vi "Has Documents.vi"(8 "error in (no error)":errorcluster, 11 "YAML Parser in":refnum<class "YAML Parser.lvclass">) -> (0 "error out":errorcluster, 3 "YAML Parser out":refnum<class "YAML Parser.lvclass">)   [LabVIEW 2015, in "YAML Parser.lvclass"]
uses:
  YAML Parser.lvclass
  <vilib>/regexp/Match Regular Expression.xnode
panel:
  out "Documents Count":i32
  out "Has Documents":bool
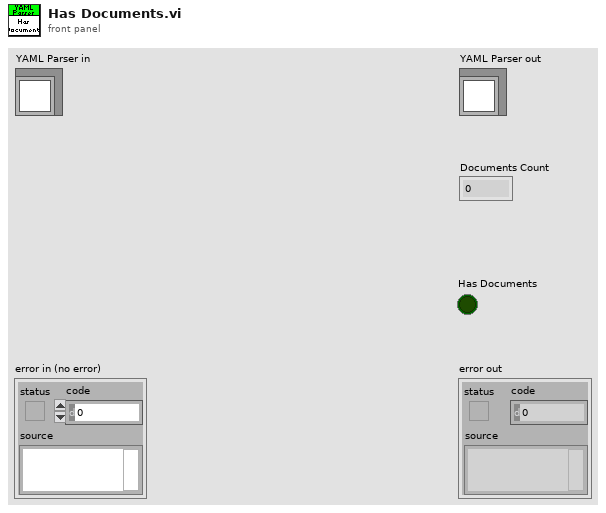
[diagram p1: front panel]
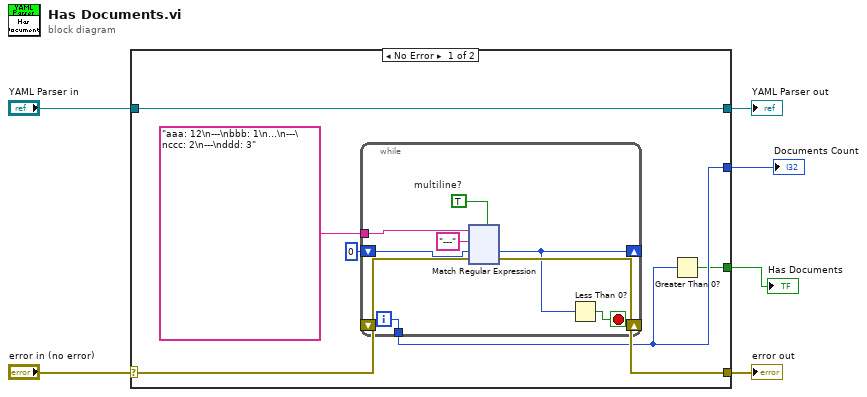
[diagram p0: block diagram]
diagram:
  n1 = case shown="No Error" "error in (no error)" {
    selector: "error in (no error)" -> [w12 w138]
    tunnel: [w11 w138] -> w5
    tunnel: [w13 w137] -> w3
    tunnel: "YAML Parser in" -> [w13 w137]
    tunnel: [w8 _] -> w2
    tunnel: [w7 _] -> w1
    frame No Error {
      n2 = while {
        tunnel: "aaa: 12\n---\nbbb: 1\n...\n---\nccc: 2\n---\nddd: 3" -> [w19]
        shift-right: [w21] -> w11
        shift-left: w12 -> [w22]
        shift-right: [w16] -> _
        shift-left: 0 ("offset past match") -> [w17]
        tunnel: [w14] -> w8
        i -> [w14]
        stop <- w15 stop-if-true
        w18 = TRUE  # multiline?
        n3 = xnode "Match Regular Expression"("input string"=w19, "regular expression"="---", "offset (0)"=w17, "error in"=w22, "multiline? (F)"=w18) -> ("offset past match"=w16:i32, "error out"=w21:errorcluster)  [unwired: 1 in, 3 out]
        n4 = Less Than 0?(x=w16) -> (x < 0?=w15:bool)
      }
      n5 = Greater Than 0?(x=w8) -> (x > 0?=w7:bool)
    }
    frame Error {
    }
  }
  "error out" <- w5
  "YAML Parser out" <- w3
  "Has Documents" <- w1
  "Documents Count" <- w2
